vi "Draw_Vertic_Lines_On_Img.vi"(6 "[IN] Color":u32(colorbox)=16711680, 8 "error IN":errorcluster, 10 "[IN] Vertical step":i32=1 min=1 max=10000 step=1, 11 "[IN] Image":T1) -> (0 "error OUT":errorcluster, 3 "[OUT] Image":T1)   [LabVIEW 2020]
uses:
  <vilib>/vision/Image Controls.llb/IMAQ Image.ctl
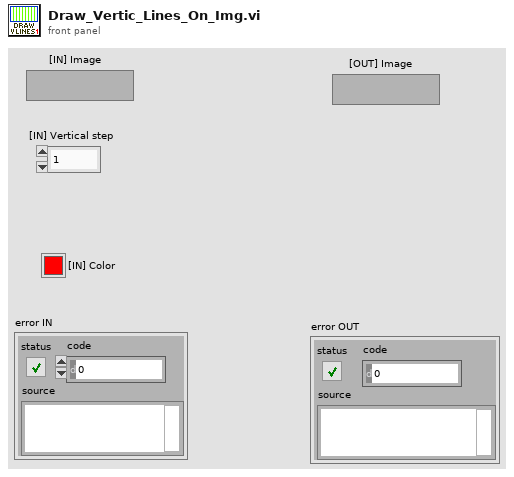
[diagram p1: front panel]
types:
  T1 = typedef "IMAQ Image.ctl" = refnum<image>
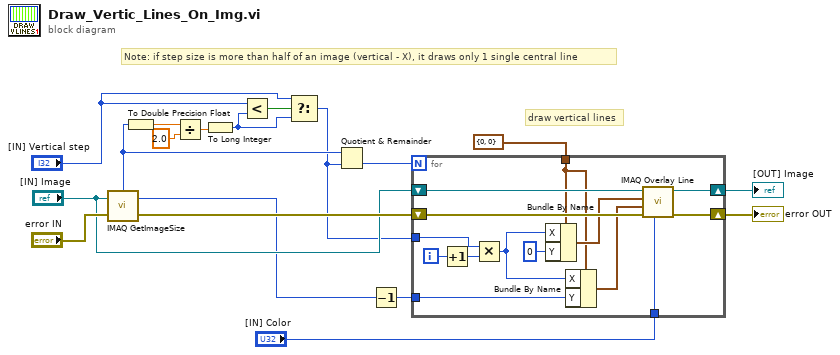
[diagram p0: block diagram]
diagram:
  # "Note: if step size is more than half of an image (vertical - X), it draws only 1 single central line"
  # "draw vertical lines"
  n1 = call "IMAQ GetImageSize"("Image"="[IN] Image", "error in (no error)"="error IN") -> ("Y Resolution"=w14:i32, "X Resolution"=w9:i32, "error out"=w17:errorcluster)  [unwired: 2 in]
  n2 = To Double Precision Float(number=w9) -> (double precision float=w8:dbl)
  n3 = Divide(x=w8, y=2.0) -> (x/y=w6:dbl)
  n4 = To Long Integer(number=w6) -> (32bit integer=w3:i32)
  n5 = Less?(x="[IN] Vertical step", y=w3) -> (x < y?=w5:bool)
  n6 = Select(t="[IN] Vertical step", s=w5, f=w3) -> (s? t:f=w2:i32)
  n7 = Quotient & Remainder(x=w9, y=w2) -> (floor(x/y)=w1:i32)  [unwired: 1 out]
  n8 = Decrement(x=w14) -> (x-1=w13:i32)
  n9 = for {
    N: w1 -> [_]
    shift-right: [w31] -> w10
    shift-left: w17 -> [w32]
    tunnel: w2 -> [w27]
    tunnel: "[IN] Color" -> [w26]
    tunnel: w13 -> [w23]
    tunnel: cluster{"X":i32, "Y":i32} {"X"=0, "Y"=0} ("Start Point") -> [w22]
    shift-right: [w19] -> w11
    shift-left: "[IN] Image" -> [w30]
    i -> [w29]
    n10 = Increment(x=w29) -> (x+1=w28:i32)
    n11 = Multiply(x=w27, y=w28) -> (x*y=w21:i32)
    n12 = Bundle By Name(cluster=w22, "X"=w21, "Y"=0) -> (w24:cluster{"X":i32, "Y":i32})
    n13 = Bundle By Name(cluster=w22, "X"=w21, "Y"=w23) -> (w20:cluster{"X":i32, "Y":i32})
    n14 = call "IMAQ Overlay Line"("Color"=w26, "error in (no error)"=w32, "End Point"=w20, "Start Point"=w24, "Image"=w30) -> ("error out"=w31:errorcluster, "Image Out"=w19:T1)  [unwired: 5 in]
  }
  "[OUT] Image" <- w11
  "error OUT" <- w10
